vi "CANFD Start Get Msg.vi"(8 "error in (no error)":errorcluster, 10 "CANIndex":u8, 11 "DevHandle":i32) -> (0 "error out":errorcluster, 3 "function return":i32)   [LabVIEW 2010, in "usb2canfd.lvlib"]
doc: "int WINAPI CANFD_StartGetMsg(int DevHandle, unsigned char CANIndex);"
uses:
  usb2canfd.lvlib
  examples/Labview/PublicFiles/USB2XXX.dll
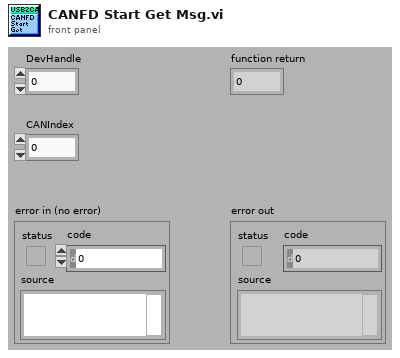
[diagram p1: front panel]
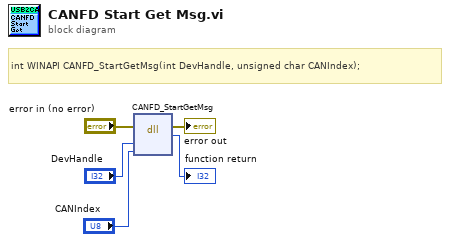
[diagram p0: block diagram]
diagram:
  # "int WINAPI CANFD_StartGetMsg(int DevHandle, unsigned char CANIndex);"
  n1 = dll-call lib="E:/OtherWork/STM32/USB2XXX_Example/examples/Labview/PublicFiles/USB2XXX.*" fn="CANFD_StartGetMsg"(error in="error in (no error)", "DevHandle"="DevHandle", "CANIndex"="CANIndex") -> (error out=→"error out":errorcluster, →"function return":i32)  [unwired: 4 in, 1 out]
